vi "AODMain.vi"   [LabVIEW 2015]
uses:
  AODControl.lvlib
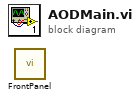
[diagram p0: block diagram]
diagram:
  n1 = call "FrontPanel.vi"() -> ()  [unwired: 12 in]
